vi "niFPGA Hanning LUT subVI.vi"(0 "address":u16, 5 "fractional index (x 2^16)":u16) -> (7 "data out":u32)   [LabVIEW 2017]
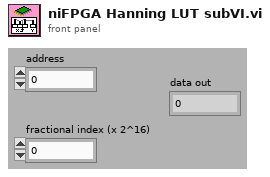
[diagram p1: front panel]
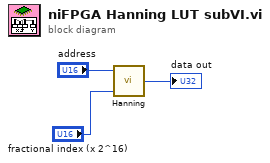
[diagram p0: block diagram]
diagram:
  n1 = call "Hanning"("address"="address", "fractional index (x 2^16)"="fractional index (x 2^16)") -> ("data out"=→"data out":u32)  [unwired: 7 in]
